vi "dynamic_tuner.vi"() -> ()   [LabVIEW 2012]
uses:
  utilities/labview/damping_freq.ctl
  calibration/dynamic_mode.ctl
  <vilib>/Platform/TimedLoop/XDataNode/timing_clust.ctl
  <vilib>/Platform/TimedLoop/XDataNode/nitl_modes.ctl
  <vilib>/Platform/TimedLoop/XDataNode/wakeup.ctl
  initialization/micron_globals.vi
  <vilib>/Platform/TimedLoop/XDataNode/XDataNode.xnode
  <vilib>/Platform/TimedLoop/XDataNode/XDNodeRunTimeDep.lvlib
panel:
  in  "Dynamic mode":T1
  in  "Save":bool
  in  "stop":bool
  in  "Store":bool
  in  "Filter":cluster{" Zeros":T2[], "Poles":T2[], "Gain":dbl}={" Zeros"=[], "Poles"=[], "Gain"=1.0} {"Gain" format="%#_3g"; "Poles"."Frequency" format="%#_3p"; "Poles"."Damping" min=0.0 max=1000.0 step=1.0 format="%#_3g"; "Zeros"."Frequency" format="%#_3p"; "Zeros"."Damping" min=0.0 max=1000.0 step=1.0 format="%#_3g"}
  in  "Load":bool
  in  "Filter file":path=path "c:/c_zz.dat"
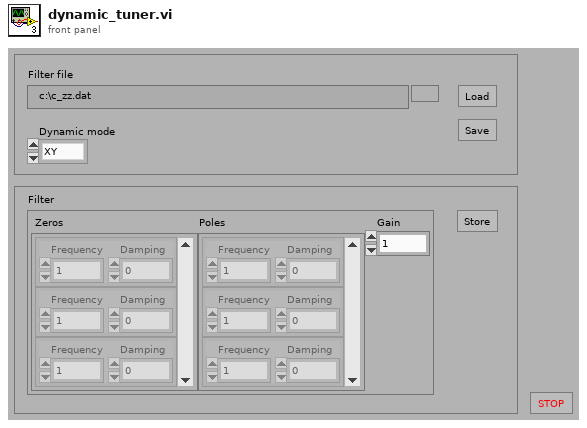
[diagram p1: front panel]
types:
  T1 = typedef "dynamic_mode.ctl" = enum16{"XY", "Rxy", "Z", "Rz"}
  T2 = typedef "damping_freq.ctl" = cluster{"Frequency":dbl, "Damping":dbl}
  T3 = typedef "ui_override_opts.ctl" = cluster{"Triggering":bool, "Parameters":bool, "Stimulus":bool, "Calibration":bool, "Modes":bool}
  T4 = typedef "XDNodeRunTimeDep.lvlib/timing_clust.ctl" = cluster{"Expected End [f-1]":u64, "Actual End [f-1]":u64, "Finished Late? [f-1]":bool, "Expected End [i-1]":u64, "Actual End [i-1]":u64, "Finished Late? [i-1]":bool, "Expected Start [i]":u64, "Actual Start [i]":u64, "Expected Start [f]":u64, "Actual Start [f]":u64, "Source Name":string, "Structure Name":string, "Period":i64, "Deadline":i64, "Offset":i64, "Start":i64, "Priority":i32, "Timeout":i32, "Mode":T5, "Wakeup Reason":T6, "Error":errorcluster, "Source Type":string, "Secondary Source Type":string, "Global End Time":u64, "Global Start Time":u64, "Frame Duration":u64, "Iteration Duration":u64, "Assigned CPU":i32, "I/O Scan Engine Mode":u32}
  T5 = typedef "XDNodeRunTimeDep.lvlib/nitl_modes.ctl" = enum32{"No Change", "Process missed periods, maintain original phase", "Discard missed periods, maintain original phase", "Process missed periods, ignore original phase", "Discard missed periods, ignore original phase"}
  T6 = typedef "XDNodeRunTimeDep.lvlib/wakeup.ctl" = enum32{"Normal", "Aborted", "Asynchronous wakeup", "Timing source error", "Timed loop error", "Timeout"}
  T7 = cluster{"filter structure":enum32{"IIR 2nd Order", "IIR 4th Order"}, "Reverse Coefficients":dbl[], "Forward Coefficients":dbl[]}
  T8 = typedef "Micron params.ctl" = cluster{"Stimulus":T9, "Goal Filter A":T11, "Mode controls":T12, "Manipulator type":enum16{"Current piezo", "Voltage piezo"}, "Manipulator calibration":T13, "Network":T15, "Goal Filter B":T11, "Cancellation":T16, "Transition time":sgl, "Estimation":T18}
  T9 = typedef "stimulus.ctl" = cluster{"Type":enum16{"Off", "Step", "Sine", "Triangle", "Arbitrary"}, "Phase":dbl, "Amplitude":sgl[], "Injection point":T10, "Closed loop":bool, "Offset":sgl[], "Tip -> world":bool, "Frequency":dbl, "Length":dbl}
  T10 = typedef "injection_point.ctl" = enum16{"Total pose", "V limiter", "Goal ", "Link position", "Link rate", "Link residue", "Link goal", "Link error", "Controller", "Output", "Drive", "DAC"}
  T11 = typedef "goal_loop_parms.ctl" = cluster{"Speedup max":sgl, "Speedup thresh":sgl, "Speedup nonlin":sgl, "Filters":cluster{"Lower Fc":sgl, "Lower Q":sgl, "Scale factor":sgl, "Upper Fc":sgl, "Upper Q":sgl, "V limit":sgl, "V limit range":sgl}[]}
  T12 = typedef "mode_conrols.ctl" = cluster{"Hold":bool, "Cancellation":bool, "Goal filter":bool, "Trigger":bool}
  T13 = typedef "manipulator_cal.ctl" = cluster{"Tool offsets":sgl[][], "Tip light calibration":T14, "Handle light calibration":T14, "Base pivots":sgl[][], "Output pivots":sgl[][], "Length center":sgl, "Workspace height":sgl[], "Workspace diameter":sgl[], "Linearization":sgl[][], "Stack travel":sgl, "Saturation pos":sgl, "Inverse filters":cluster{"filter structure":enum32{"IIR 2nd Order", "IIR 4th Order"}, "Reverse Coefficients":dbl[], "Forward Coefficients":dbl[]}[]}
  T14 = typedef "probe_calibration.ctl" = sgl[][]
  T15 = typedef "network_params.ctl" = cluster{"Remote Host":string, "Send Status":bool, "Send Port":u16, "Recv Commands":bool, "Recv Port":u16}
  T16 = typedef "sq_control_params.ctl" = cluster{"KP":T17, "KI":sgl, "KD":T17, "Max vel":sgl, "Max acc":sgl, "Int error limit":sgl, "RCM gain":sgl, "Bypass":bool}
  T17 = typedef "decoupled_gain.ctl" = cluster{"XY":sgl, "Rxy":sgl, "Z":sgl, "Rz":sgl}
  T18 = typedef "estimation_controls.ctl" = cluster{"Link":cluster{"Measure noise":dbl[], "Process noise":dbl[], "Innovation limit":dbl[], "Enable":bool}, "Handle":cluster{"Measure noise":dbl[], "Process noise":dbl[], "State limits":dbl[], "Innovation limit":dbl[], "Prediction Lookahead":sgl, "Enable":bool}}
  T19 = cluster{"filter structure":enum32{"IIR 2nd Order", "IIR 4th Order"}, "Reverse Coefficients":dbl[], "Forward Coefficients":dbl[]}[]
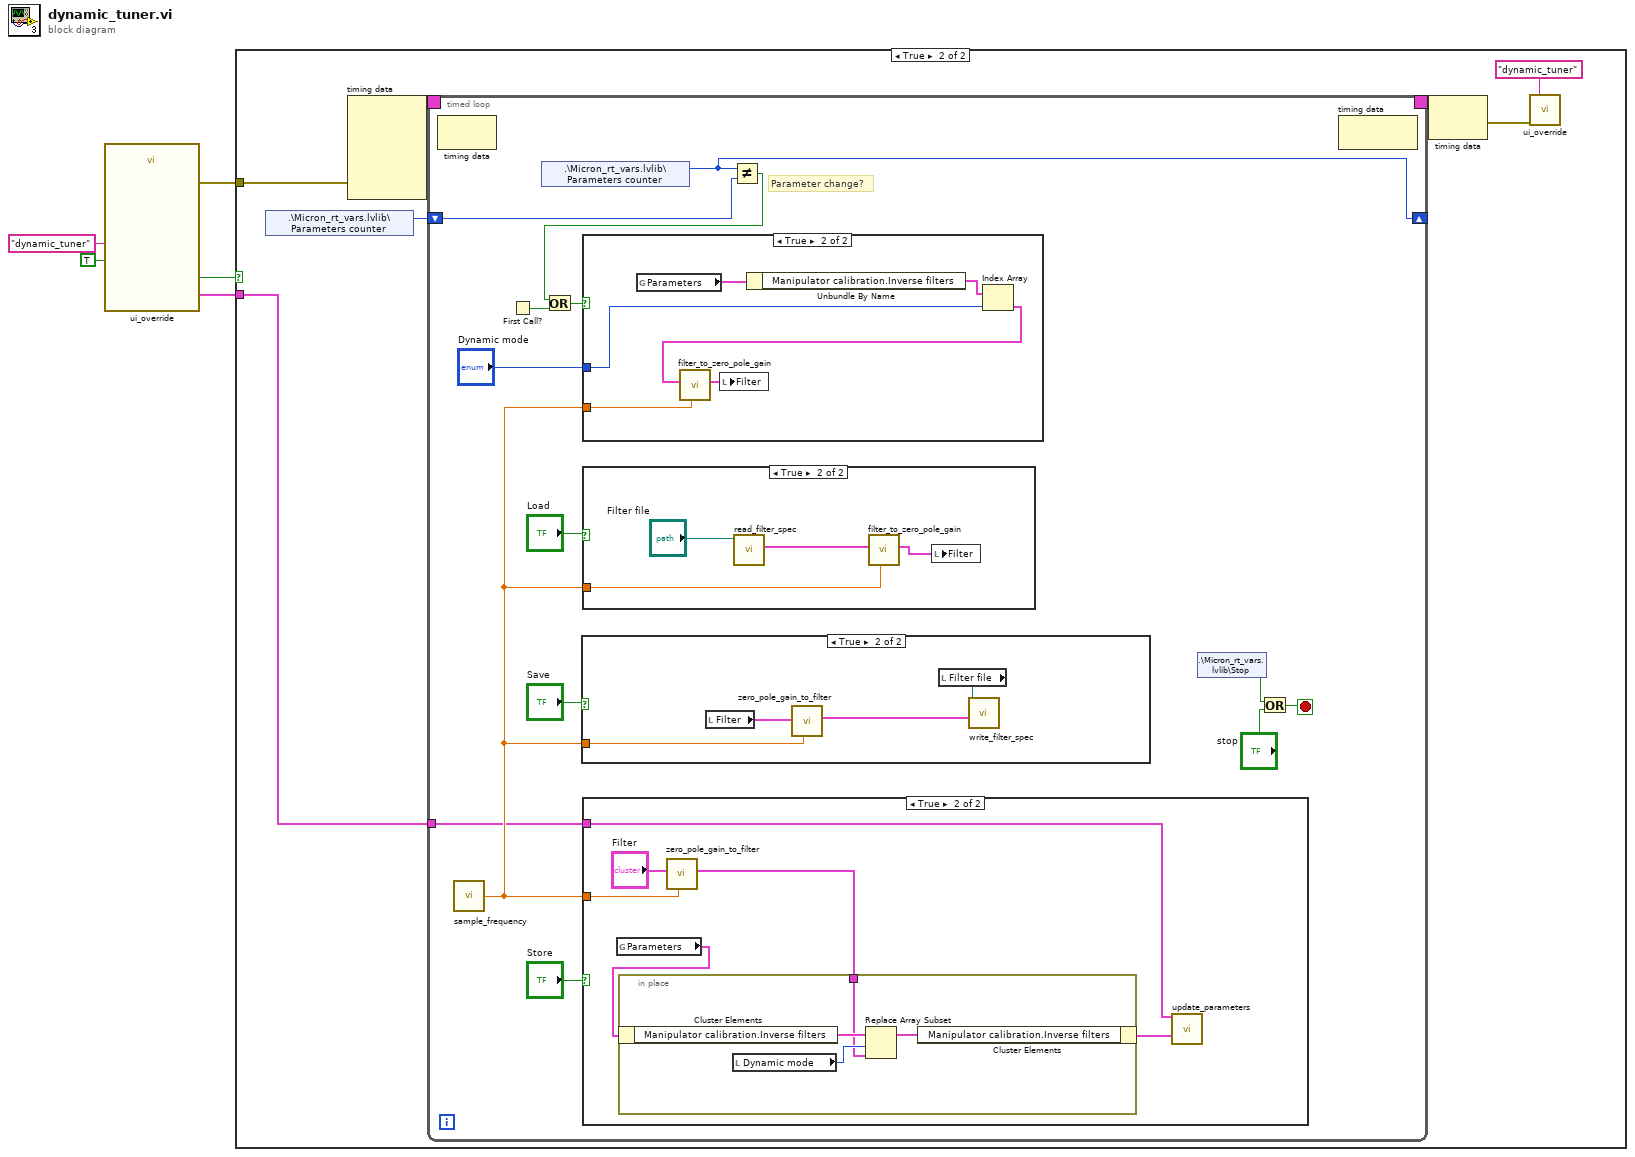
[diagram p0: block diagram]
diagram:
  n1 = call "ui_override.vi"("VI name"="dynamic_tuner", "Calibration"=TRUE) -> ("Override"=w1:T3, "Got all"=w2:bool, "error out"=w5:errorcluster)  [unwired: 11 in]
  n2 = case shown="True" w2 {
    tunnel: w5 -> [_ w9]
    tunnel: w1 -> [_ w8]
    frame False {
    }
    frame True {
      n3 = shared-variable ".\\Micron_rt_vars.lvlib\\Parameters counter"() -> (w10:u32)  [unwired: 2 out]
      n4 = node-c288(w9) -> (w12:T4)  [unwired: 4 out]
      n5 = timed-loop {
        timing: w12 -> [_]
        timing-out: [_] -> w11
        shift-right: [w23] -> _
        shift-left: w10 -> [w24]
        tunnel: w8 -> [w16]
        stop <- w15 stop-if-true
        # "Parameter change?"
        n6 = node-c288() -> ()  [unwired: 2 out]
        n7 = call "sample_frequency.vi"() -> ("Sample frequency"=w18:dbl)
        n8 = First Call?() -> (First Call?: T/F=w21:bool)
        n9 = shared-variable ".\\Micron_rt_vars.lvlib\\Parameters counter"() -> (w23:u32)  [unwired: 2 out]
        n10 = case shown="True" "Save" {
          tunnel: w18 -> [_ w28]
          frame False {
          }
          frame True {
            n11 = local read "Filter"() -> (w29:cluster{" Zeros":T2[], "Poles":T2[], "Gain":dbl})
            n12 = call "zero_pole_gain_to_filter.vi"("Fs"=w28, "Zero/Pole/Gain"=w29) -> ("IIR Filter Cluster"=w27:T7)  [unwired: 9 out]
            n13 = local read "Filter file"() -> (w30:path)
            n14 = call "write_filter_spec.vi"("IIR Filter Cluster"=w27, "File path"=w30) -> ()  [unwired: 9 in, 1 out]
          }
        }
        n15 = case shown="True" "Load" {
          tunnel: w18 -> [_ w47]
          frame False {
          }
          frame True {
            n16 = call "read_filter_spec.vi"("File path"="Filter file") -> ("IIR Filter Cluster"=w48:T7)  [unwired: 10 out]
            n17 = call "filter_to_zero_pole_gain.vi"("Fs"=w47, "IIR Filter Cluster"=w48) -> ("Zero/Pole/Gain"=w49:cluster{" Zeros":T2[], "Poles":T2[], "Gain":dbl})  [unwired: 9 out]
            n18 = local write "Filter"(w49) -> ()
          }
        }
        n19 = case shown="True" "Store" {
          tunnel: w18 -> [_ w35]
          tunnel: w16 -> [_ w34]
          frame False {
          }
          frame True {
            n20 = global read "micron_globals.vi" "Parameters"() -> (w33:T8)
            n21 = call "zero_pole_gain_to_filter.vi"("Fs"=w35, "Zero/Pole/Gain"="Filter") -> ("IIR Filter Cluster"=w32:T7)  [unwired: 9 out]
            n22 = in-place {
              in-place-border: w32 -> [w38]
              n23 = in-place-cluster #1(w33) -> ("Manipulator calibration.Inverse filters"=w40:T19)
              n24 = local read "Dynamic mode"() -> (w39:T1)
              n25 = Replace Array Subset(array=w40, new element=w38, index=w39) -> (w37:T19)
              n26 = in-place-cluster #1("Manipulator calibration.Inverse filters"=w37) -> (w31:T8)
            }
            n27 = call "update_parameters.vi"("Modify"=w34, "Parameters"=w31) -> ()  [unwired: 12 in, 2 out]
          }
        }
        n28 = Not Equal?(x=w23, y=w24) -> (x != y?=w20:bool)
        n29 = Or(x=w20, y=w21) -> (x .or. y?=w22:bool)
        n30 = case shown="True" w22 {
          tunnel: w18 -> [_ w44]
          tunnel: "Dynamic mode" -> [_ w42]
          frame False {
          }
          frame True {
            n31 = global read "micron_globals.vi" "Parameters"() -> (w45:T8)
            n32 = Unbundle By Name(w45) -> ("Manipulator calibration.Inverse filters"=w43:T19)
            n33 = Index Array(array=w43, index=w42) -> (element=w41:T7)
            n34 = call "filter_to_zero_pole_gain.vi"("Fs"=w44, "IIR Filter Cluster"=w41) -> ("Zero/Pole/Gain"=w46:cluster{" Zeros":T2[], "Poles":T2[], "Gain":dbl})  [unwired: 9 out]
            n35 = local write "Filter"(w46) -> ()
          }
        }
        n36 = shared-variable ".\\Micron_rt_vars.lvlib\\Stop"() -> (w14:bool)  [unwired: 1 in, 1 out]
        n37 = Or(x=w14, y="stop") -> (x .or. y?=w15:bool)
        n38 = node-c288() -> ()  [unwired: 2 out]
      }
      n39 = node-c288(w11) -> (w7:errorcluster)
      n40 = call "ui_override.vi"("VI name"="dynamic_tuner", "error in"=w7) -> ()  [unwired: 11 in, 3 out]
    }
  }
